vi "计算.vi"(8 "error in (no error)":errorcluster caption="错误输入（无错误）", 11 "减法类 输入":refnum<class "减法类.lvclass"> caption="DNL_LabVIEW Object in") -> (0 "error out":errorcluster caption="错误输出", 2 "结果":dbl, 3 "减法类 输出":refnum<class "减法类.lvclass"> caption="DNL_LabVIEW Object out")   [LabVIEW 2013, in "减法类.lvclass"]
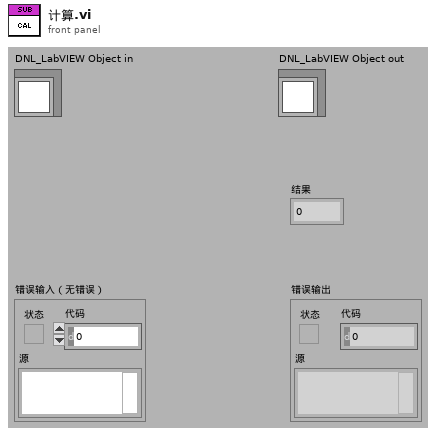
[diagram p1: front panel]
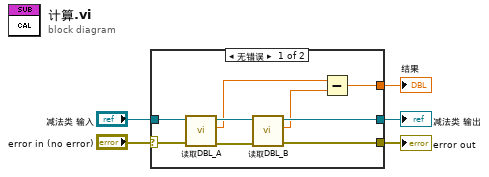
[diagram p0: block diagram]
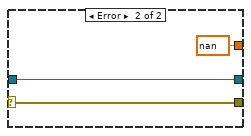
[diagram p2: hidden frame]
diagram:
  n1 = case shown="无错误" "error in (no error)" {
    selector: "error in (no error)" -> [w14 w17]
    tunnel: [w12 w17] -> w4
    tunnel: "减法类 输入" -> [w11 w16]
    tunnel: [w9 w16] -> w2
    tunnel: [w6 nan] -> w1
    frame No Error {
      n2 = call "读取DBL_A.vi"("error in (no error)"=w14, "运算类输入"=w11) -> ("error out"=w13:errorcluster, "DBL_A"=w8:dbl, "运算类输出"=w10:refnum<class "减法类.lvclass">)  [unwired: 7 in]
      n3 = call "读取DBL_B.vi"("error in (no error)"=w13, "运算类输入"=w10) -> ("error out"=w12:errorcluster, "DBL_B"=w7:dbl, "运算类输出"=w9:refnum<class "减法类.lvclass">)  [unwired: 7 in]
      n4 = Subtract(x=w8, y=w7) -> (x-y=w6:dbl)
    }
    frame Error {
    }
  }
  "结果" <- w1
  "error out" <- w4
  "减法类 输出" <- w2
